vi "11.2.2.-Momento Invariante de Hu Inicial - Mpq.vi"(9 "f":dbl[][](array[numeric]), 10 "Y":dbl[][](array[numeric]), 11 "X":dbl[][](array[numeric])) -> (1 "mpq10":dbl, 2 "xc":dbl, 3 "mpq00":dbl, 4 "yc":dbl, 5 "mpq01":dbl)   [LabVIEW 2020]
panel:
  # "Visión Artificial - Momentos Invariantes de Hu\nDiego Cervantes Rodríguez\ndicer0.com"
  # "Momento inicial = Mpq = sum(sum((x^p)*(y^q)*f(x,y)))"
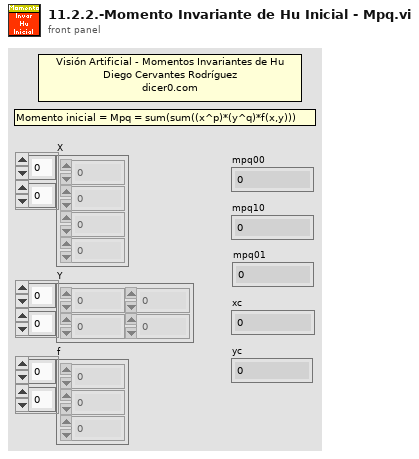
[diagram p1: front panel]
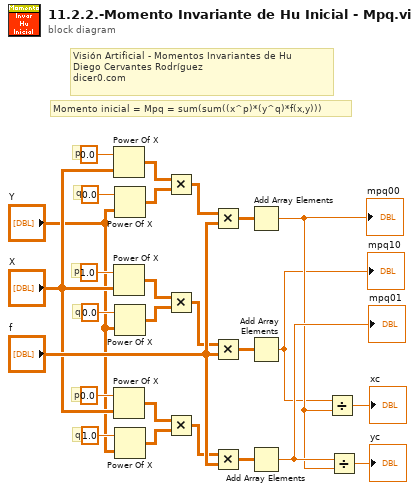
[diagram p0: block diagram]
diagram:
  # "Momento inicial = Mpq = sum(sum((x^p)*(y^q)*f(x,y)))"
  # "Visión Artificial - Momentos Invariantes de Hu\nDiego Cervantes Rodríguez\ndicer0.com"
  # "p"
  # "q"
  # "p"
  # "q"
  # "q"
  # "p"
  n1 = Power Of X(1:"X", 2:0.0) -> (0:w5:dbl[][])
  n2 = Power Of X(1:"X", 2:1.0) -> (0:w11:dbl[][])
  n3 = Power Of X(1:"X", 2:0.0) -> (0:w17:dbl[][])
  n4 = Power Of X(1:"Y", 2:0.0) -> (0:w6:dbl[][])
  n5 = Power Of X(1:"Y", 2:0.0) -> (0:w12:dbl[][])
  n6 = Power Of X(1:"Y", 2:1.0) -> (0:w18:dbl[][])
  n7 = Multiply(x=w5, y=w6) -> (x*y=w7:dbl[][])
  n8 = Multiply(x=w11, y=w12) -> (x*y=w13:dbl[][])
  n9 = Multiply(x=w17, y=w18) -> (x*y=w19:dbl[][])
  n10 = Multiply(x=w7, y="f") -> (x*y=w8:dbl[][])
  n11 = Multiply(x=w13, y="f") -> (x*y=w14:dbl[][])
  n12 = Multiply(x=w19, y="f") -> (x*y=w20:dbl[][])
  n13 = Add Array Elements(numeric array=w8) -> (sum=w23:dbl)
  "mpq00" <- w23
  n14 = Add Array Elements(numeric array=w14) -> (sum=w22:dbl)
  "mpq10" <- w22
  n15 = Add Array Elements(numeric array=w20) -> (sum=w24:dbl)
  "mpq01" <- w24
  n16 = Divide(x=w22, y=w23) -> (x/y=→"xc":dbl)
  n17 = Divide(x=w24, y=w23) -> (x/y=→"yc":dbl)
